vi "2_10.vi"() -> ()   [LabVIEW 2015]
panel:
  out "Multiplication Table":dbl[](array[numeric])
  in  "Number":i8
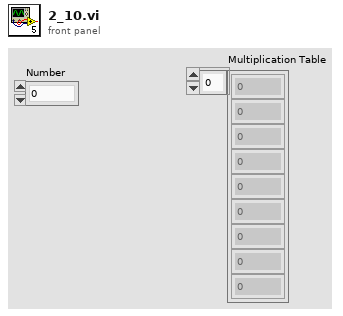
[diagram p1: front panel]
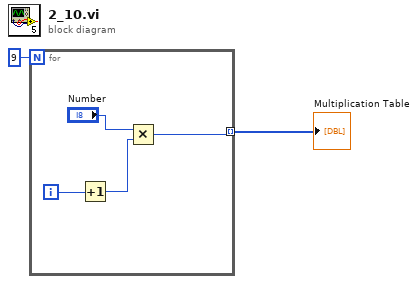
[diagram p0: block diagram]
diagram:
  n1 = for {
    N: 9 -> [_]
    tunnel: [w3] -> w1 mode=indexing
    i -> [w5]
    n2 = Increment(x=w5) -> (x+1=w4:i32)
    n3 = Multiply(x="Number", y=w4) -> (x*y=w3:i32)
  }
  "Multiplication Table" <- w1
